vi "Create Mesh Grid (2D).vi"   [LabVIEW 2020, in "NI_Gmath.lvlib"]
doc: "Takes two <B>x domain</B> and <B>y domain</B> arrays and forms <B>X</B> and <B>Y</B> 2D arrays, which are typically used to evaluate and plot functions of two variables. You must manually select the polymorphic instance to use."
uses:
  NI_Gmath.lvlib
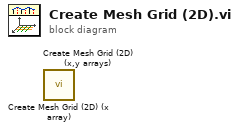
[diagram p0: block diagram]
diagram:
  n1 = call "Create Mesh Grid (2D) (x array).vi"() -> ()  [unwired: 9 in, 3 out]
  n2 = call "Create Mesh Grid (2D) (x,y arrays).vi"() -> ()  [unwired: 9 in, 3 out]
